vi "datatofile 2c.vi"(5 "A2":dbl[](array[numeric]), 7 "A1":dbl[](array[numeric]), 8 "error in":errorcluster, 10 "title":string="No data\n", 11 "file path (dialog if empty)":path=path "C:/LabView/Guang Yue lab view learning/data/temp.txt") -> (0 "error out":errorcluster)   [LabVIEW 2024]
uses:
  <vilib>/Utility/file.llb/Write Delimited Spreadsheet (DBL).vi
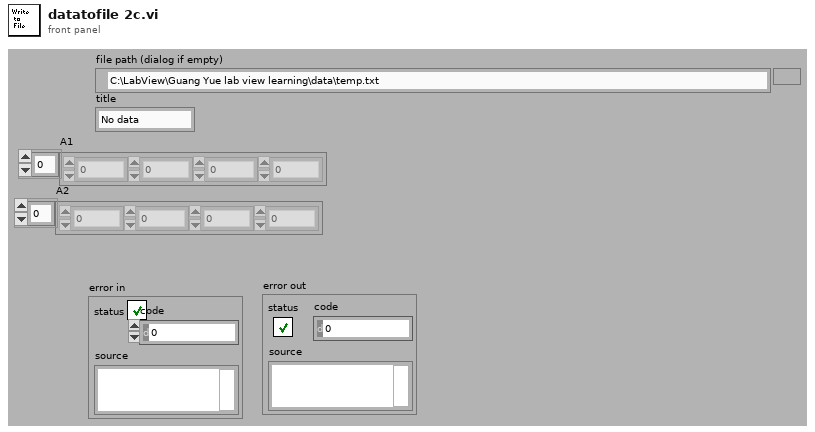
[diagram p1: front panel]
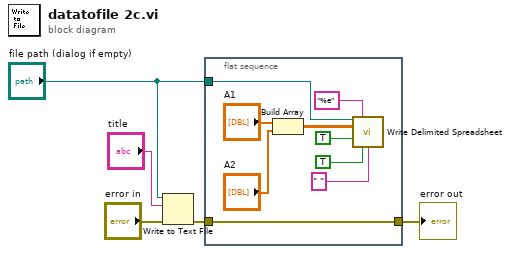
[diagram p0: block diagram]
diagram:
  n1 = Write to Text File(file (use dialog)="file path (dialog if empty)", text="title", error in="error in") -> (error out=w1:errorcluster)  [unwired: 1 in, 2 out]
  n2 = flat-sequence {
    tunnel: "file path (dialog if empty)" -> [w10]
    tunnel: [w14] -> w2
    tunnel: w1 -> [w14]
    frame #0 {
      n3 = Build Array("A1", "A2") -> (w11:dbl[][])
      n4 = call-poly <vilib>:"Write Delimited Spreadsheet.vi"("file path (dialog if empty)"=w10, "format (%.3f)"="%e", "2D data"=w11, "append to file? (new file:F)"=TRUE, "transpose? (no:F)"=TRUE, "delimiter (\\t)"=" " ("delimiter (\\t)")) -> ()  [unwired: 8 in, 2 out]
    }
  }
  "error out" <- w2
